vi "RT.vi"() -> ()   [LabVIEW 2013]
uses:
  <vilib>/Platform/TimedLoop/XDataNode/timing_clust.ctl
  <vilib>/Platform/TimedLoop/XDataNode/nitl_modes.ctl
  <vilib>/Platform/TimedLoop/XDataNode/wakeup.ctl
  <vilib>/Platform/TimedLoop/XDataNode/loadnilvce.vi
  <vilib>/platform/TimedLoop/XDataNode/XDataNode.xnode
  <vilib>/Platform/TimedLoop/XDataNode/XDNodeRunTimeDep.lvlib
  <vilib>/ptbypt/NI_PtbyPt.lvlib
panel:
  in  "Stop Button":bool
  out "Temperature":T1(graph)
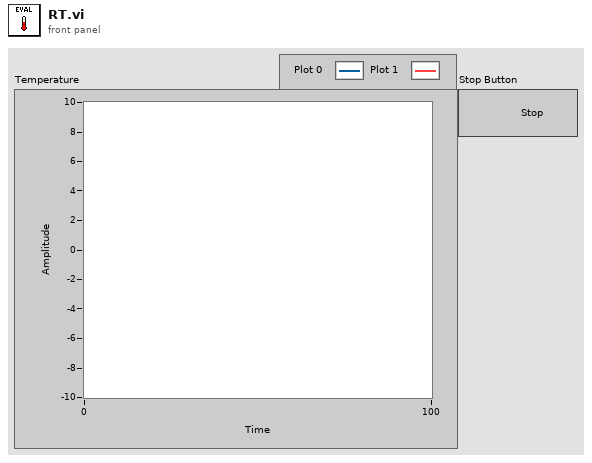
[diagram p1: front panel]
types:
  T1 = cluster{"Array of Double[0]":dbl, "Array of Double[1]":dbl, "Array of Double[2]":dbl, "Array of Double[3]":dbl, "Array of Double[4]":dbl, "Array of Double[5]":dbl, "Array of Double[6]":dbl, "Array of Double[7]":dbl, "Array of Double[8]":dbl}
  T2 = typedef "XDNodeRunTimeDep.lvlib/timing_clust.ctl" = cluster{"Expected End [f-1]":u64, "Actual End [f-1]":u64, "Finished Late? [f-1]":bool, "Expected End [i-1]":u64, "Actual End [i-1]":u64, "Finished Late? [i-1]":bool, "Expected Start [i]":u64, "Actual Start [i]":u64, "Expected Start [f]":u64, "Actual Start [f]":u64, "Source Name":string, "Structure Name":string, "Period":i64, "Deadline":i64, "Offset":i64, "Start":i64, "Priority":i32, "Timeout":i32, "Mode":T3, "Wakeup Reason":T4, "Error":errorcluster, "Source Type":string, "Secondary Source Type":string, "Global End Time":u64, "Global Start Time":u64, "Frame Duration":u64, "Iteration Duration":u64, "Assigned CPU":i32, "I/O Scan Engine Mode":u32}
  T3 = typedef "XDNodeRunTimeDep.lvlib/nitl_modes.ctl" = enum32{"No Change", "Process missed periods, maintain original phase", "Discard missed periods, maintain original phase", "Process missed periods, ignore original phase", "Discard missed periods, ignore original phase"}
  T4 = typedef "XDNodeRunTimeDep.lvlib/wakeup.ctl" = enum32{"Normal", "Aborted", "Asynchronous wakeup", "Timing source error", "Timed loop error", "Timeout"}
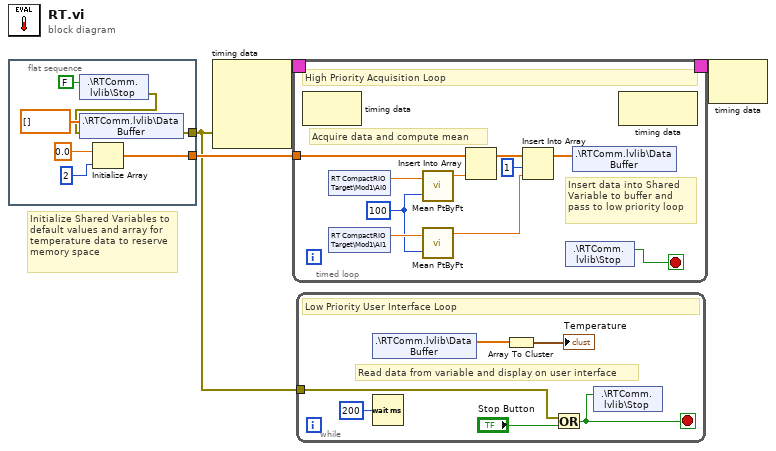
[diagram p0: block diagram]
diagram:
  # "Initialize Shared Variables to\ndefault values and array for \ntemperature data to reserve\nmemory space"
  n1 = flat-sequence {
    tunnel: [w7] -> w2
    tunnel: [w5] -> w1
    frame #0 {
      n2 = shared-variable ".\\RTComm.lvlib\\Stop"(FALSE ("Stop")) -> (error out=w6:errorcluster)  [unwired: 1 in]
      n3 = shared-variable ".\\RTComm.lvlib\\Data Buffer"(dbl[] [] ("Data Buffer"), error in=w6) -> (error out=w5:errorcluster)
      n4 = Initialize Array(0.0 ("AI3"), 2 ("dimension size")) -> (w7:dbl[])
    }
  }
  n5 = node-c288(w1) -> (w4:T2)  [unwired: 3 in]
  n6 = timed-loop {
    timing: w4 -> [_]
    timing-out: [_] -> w3
    tunnel: w2 -> [w19]
    stop <- w21 stop-if-true
    w16 = 100 ("sample length")
    # "Insert data into Shared \nVariable to buffer and \npass to low priority loop"
    # "Acquire data and compute mean"
    # "High Priority Acquisition Loop"
    n7 = node-c288() -> ()  [unwired: 1 in, 1 out]
    n8 = shared-variable "RT CompactRIO Target\\Mod1\\AI0"() -> (w20:dbl)  [unwired: 1 in, 1 out]
    n9 = shared-variable "RT CompactRIO Target\\Mod1\\AI1"() -> (w17:dbl)  [unwired: 1 in, 1 out]
    n10 = call <vilib>:"Mean PtByPt.vi"("x"=w20, "sample length"=w16) -> ("mean"=w18:dbl)  [unwired: 2 in, 1 out]
    n11 = call <vilib>:"Mean PtByPt.vi"("x"=w17, "sample length"=w16) -> ("mean"=w13:dbl)  [unwired: 2 in, 1 out]
    n12 = Insert Into Array(array=w19, new element=w18) -> (w15:dbl[])  [unwired: 1 in]
    n13 = Insert Into Array(array=w15, index=1, new element=w13) -> (w14:dbl[])
    n14 = shared-variable ".\\RTComm.lvlib\\Stop"() -> (w21:bool)  [unwired: 1 in, 1 out]
    n15 = shared-variable ".\\RTComm.lvlib\\Data Buffer"(w14) -> ()  [unwired: 1 in, 1 out]
    n16 = node-c288() -> ()  [unwired: 1 in, 1 out]
  }
  n17 = while {
    tunnel: w1 -> [w24]
    stop <- w25 stop-if-true
    # "Read data from variable and display on user interface"
    # "Low Priority User Interface Loop"
    n18 = shared-variable ".\\RTComm.lvlib\\Data Buffer"() -> (w28:dbl[])  [unwired: 1 in, 1 out]
    n19 = Wait (ms)(milliseconds to wait=u32 200) -> ()  [unwired: 1 out]
    n20 = Array To Cluster(array=w28) -> (cluster=→"Temperature":T1)
    n21 = Or(x=w24, y="Stop Button") -> (x .or. y?=w25:bool)
    n22 = shared-variable ".\\RTComm.lvlib\\Stop"(w25) -> ()  [unwired: 1 in, 1 out]
  }
  n23 = node-c288(w3) -> ()  [unwired: 1 out]
